vi "Get Shared Memory Size.vi"(8 "error in (no error)":errorcluster, 11 "shared memory in":T1) -> (0 "error out":errorcluster, 2 "size (bytes)":u64, 3 "shared memory out":T1)   [LabVIEW 2013, in "Linux RT IPC.Shared Memory.lvlib" / "Shared Memory.lvclass"]
doc: "This VI returns the current size in bytes of the shared memory file."
uses:
  Shared Memory.lvclass
  Controls/reference.ctl
  Shared Memory.lvclass/Shared Memory.ctl
  Linux RT IPC.Shared Memory.lvlib
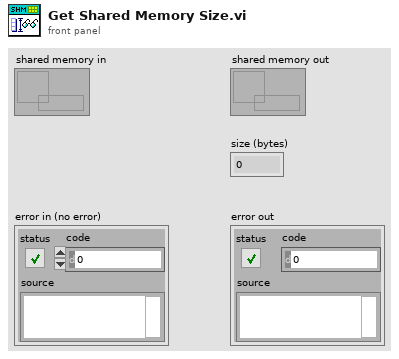
[diagram p1: front panel]
types:
  T1 = typedef "Linux RT IPC.Shared Memory.lvlib/reference.ctl" = refnum<data-value>
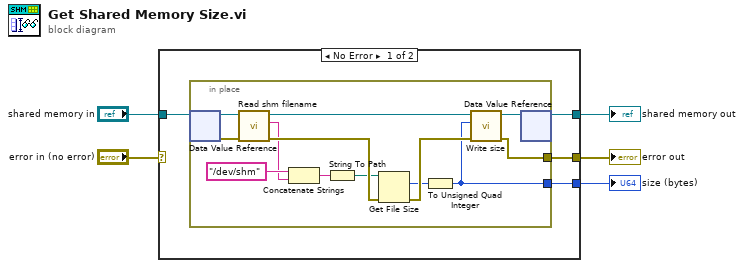
[diagram p0: block diagram]
diagram:
  n1 = case shown="No Error" "error in (no error)" {
    selector: "error in (no error)" -> [_ w23]
    tunnel: "shared memory in" -> [w9 w24]
    tunnel: [w8 w23] -> w2
    tunnel: [w7 w24] -> w4
    tunnel: [w6 _] -> w1
    frame No Error {
      n2 = in-place {
        in-place-border: [w19] -> w8
        in-place-border: [w10] -> w6
        n3 = in-place-dvr #1(w9) -> (w22:refnum<class "Shared Memory.lvclass">, w20:errorcluster)
        n4 = call "Read shm filename.vi"("error in (no error)"=w20, "Shared Memory in"=w22) -> ("error out"=w18:errorcluster, "shm filename"=w12:string, "Shared Memory out"=w16:refnum<class "Shared Memory.lvclass">)  [unwired: 7 in]
        n5 = Concatenate Strings("/dev/shm", w12) -> (w14:string)
        n6 = String To Path(string=w14) -> (path=w13:path)
        n7 = Get File Size(file=w13, error in=w18) -> (size (in bytes)=w11:i64, 0:w17:errorcluster)  [unwired: 1 out]
        n8 = To Unsigned Quad Integer(1:w11) -> (0:w10:u64)
        n9 = call "Write size.vi"("error in (no error)"=w17, "size (bytes)"=w10, "Shared Memory in"=w16) -> ("error out"=w19:errorcluster, "Shared Memory out"=w21:refnum<class "Shared Memory.lvclass">)  [unwired: 7 in]
        n10 = in-place-dvr #1(w21) -> (w7:T1)  [unwired: 1 out]
      }
    }
    frame Error {
    }
  }
  "size (bytes)" <- w1
  "error out" <- w2
  "shared memory out" <- w4
